vi "Untitled 1.vi"() -> ()   [LabVIEW 2020]
panel:
  in  "stop":bool
  in  "Vertical Pointer Slide":dbl(slide) scale=0.0..10.0
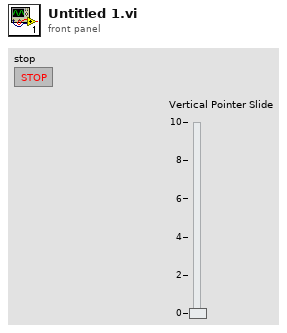
[diagram p1: front panel]
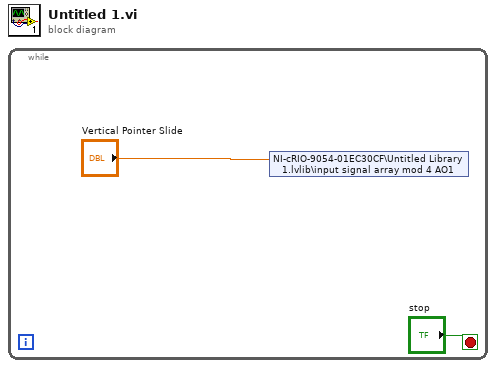
[diagram p0: block diagram]
diagram:
  n1 = while {
    stop <- "stop" stop-if-true
    n2 = shared-variable "NI-cRIO-9054-01EC30CF\\Untitled Library 1.lvlib\\input signal array mod 4 AO1"("Vertical Pointer Slide") -> ()  [unwired: 1 in, 1 out]
  }
